vi "Chronos TDMS Add Data to Plot.vi"(8 "data":dbl[][](array[numeric]), 9 "Ch Names":string[](array[string]), 10 "plot names in":string[](array[string]), 11 "XY Graph in":cluster{dbl[], dbl[]}[](graph)) -> (1 "end time":dbl, 2 "plot names out":string[](array[string]), 3 "XY Graph":cluster{dbl[], dbl[]}[](graph))   [LabVIEW 2021]
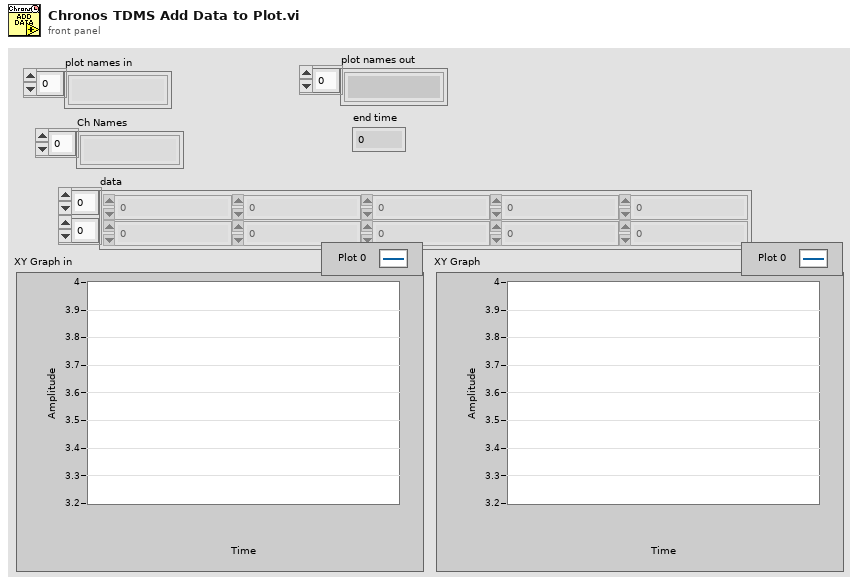
[diagram p1: front panel]
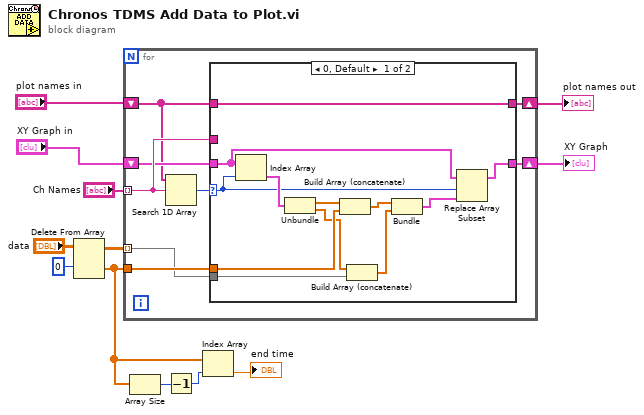
[diagram p0: block diagram]
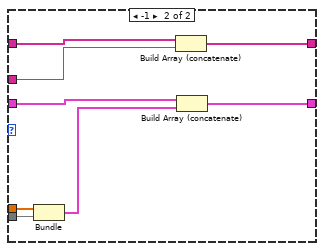
[diagram p2: hidden frame]
diagram:
  n1 = Delete From Array(array="data", index (row)=0) -> (deleted portion=w4:dbl[], array with subset deleted=w11:dbl[][])  [unwired: 2 in]
  n2 = for {
    tunnel: w11 -> [w19] mode=indexing
    tunnel: w4 -> [w20]
    tunnel: "Ch Names" -> [w17] mode=indexing
    shift-right: [w16] -> w6
    shift-left: "plot names in" -> [w13]
    shift-right: [w15] -> w5
    shift-left: "XY Graph in" -> [w14]
    n3 = Search 1D Array(1D array=w13, element=w17) -> (index of element=w18:i32)  [unwired: 1 in]
    n4 = case shown="0, Default" w18 {
      selector: w18 -> [w24 _]
      tunnel: w20 -> [w29 w40]
      tunnel: w19 -> [w28 w39]
      tunnel: w17 -> [_ w38]
      tunnel: [w32 w36] -> w16
      tunnel: w13 -> [w32 w35]
      tunnel: [w21 w34] -> w15
      tunnel: w14 -> [w22 w33]
      frame 0, Default {
        n5 = Index Array(array=w22, index=w24) -> (element=w31:cluster{dbl[], dbl[]})
        n6 = Unbundle(w31) -> (w30:dbl[], w27:dbl[])
        n7 = Build Array (concatenate)(w30, w29) -> (w26:dbl[])
        n8 = Build Array (concatenate)(w27, w28) -> (w25:dbl[])
        n9 = Bundle(w26, w25) -> (w23:cluster{dbl[], dbl[]})  [unwired: 1 in]
        n10 = Replace Array Subset(array=w22, new element=w23, index=w24) -> (w21:cluster{dbl[], dbl[]}[])
      }
      frame -1 {
        n11 = Bundle("data"=w40, "data"=w39) -> (w37:cluster{"data":dbl[], "data":dbl[]})  [unwired: 1 in]
        n12 = Build Array (concatenate)(w35, w38) -> (w36:string[])
        n13 = Build Array (concatenate)(w33, w37) -> (w34:cluster{"data":dbl[], "data":dbl[]}[])
      }
    }
  }
  "XY Graph" <- w5
  "plot names out" <- w6
  n14 = Array Size(array=w4) -> (size(s)=w3:i32)
  n15 = Decrement(x=w3) -> (x-1=w2:i32)
  n16 = Index Array(array=w4, index=w2) -> (element=→"end time":dbl)
